vi "Send Set Polling Message.vi"(8 "error in (no error)":errorcluster, 10 "Polling Message":refnum<class "Message.lvclass">, 11 "Message Queue in":refnum<queue>) -> (0 "error out":errorcluster, 3 "Message Queue out":refnum<queue>)   [LabVIEW 2024, in "OOQMH.lvlib" / "Set Polling Message.lvclass"]
uses:
  Set Polling Message.lvclass
  Set Polling Message.lvclass/Set Polling Message.ctl
  C:/Users/uspoaotto/OneDrive - Oregon Tool/Desktop/working copies/helperLoop/src/OOQMH/Message/Message.lvclass
  C:/Users/uspoaotto/OneDrive - Oregon Tool/Desktop/working copies/helperLoop/src/OOQMH/Set Polling Message/Set Polling Message.lvclass
  Message/Message.lvclass
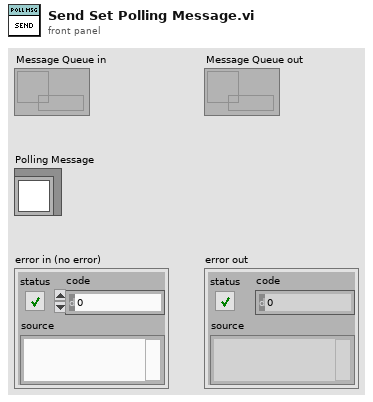
[diagram p1: front panel]
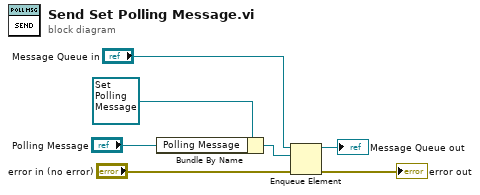
[diagram p0: block diagram]
diagram:
  n1 = Bundle By Name(cluster=refnum<class "Set Polling Message.lvclass"> refnum ("OOQMH.lvlib:Set Polling Message.lvclass"), "Polling Message"="Polling Message") -> (w5:refnum<class "Set Polling Message.lvclass">)
  n2 = Enqueue Element(queue="Message Queue in", element=w5, error in (no error)="error in (no error)") -> (queue out=→"Message Queue out":refnum<queue>, error out=→"error out":errorcluster)  [unwired: 1 in, 1 out]
